vi "Read TopicLookupTable.vi"(11 "Mediator in":refnum<class "Mediator.lvclass">) -> (2 "TopicLookupTable":refnum<data-value>)   [LabVIEW 2020, in "Mediator.lvlib" / "Mediator.lvclass"]
uses:
  <vilib>/gpm_packages/@cs/mva-core/Source/Mediator/Mediator/Mediator.lvclass
  <vilib>/gpm_packages/@cs/mva-core/Source/Mediator/TopicLookupTable/TopicLookupTable.lvclass
  <vilib>/gpm_packages/@cs/mva-core/Source/Mediator/Mediator/Mediator.lvclass/Mediator.ctl
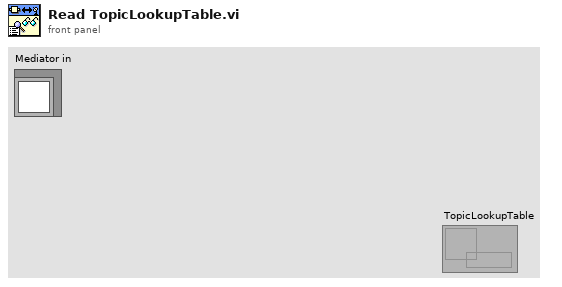
[diagram p1: front panel]
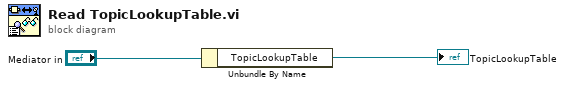
[diagram p0: block diagram]
diagram:
  n1 = Unbundle By Name("Mediator in") -> ("TopicLookupTable"=→"TopicLookupTable":refnum<data-value>)
